vi "Test Case Description Reset on Test Start.vi"(8 "error in (no error)":errorcluster, 11 "Result Model Result Recording Test in":refnum<class "Result Model Result Recording Test.lvclass">) -> (0 "error out":errorcluster, 3 "Result Model Result Recording Test out":refnum<class "Result Model Result Recording Test.lvclass">)   [LabVIEW 2020, in "Result Model Result Recording Test.lvclass"]
uses:
  Result Model Result Recording Test.lvclass
  source/Core/Result/Type.ctl
  source/Core/Result/Result.lvlib
  source/Core/Result/Status.ctl
  source/Core/Result/Result.ctl
  ae2c71b8-32bb-49d1-8500-0119bfec74ff.vi
  source/User Interface/Result Model/Result Model.lvclass
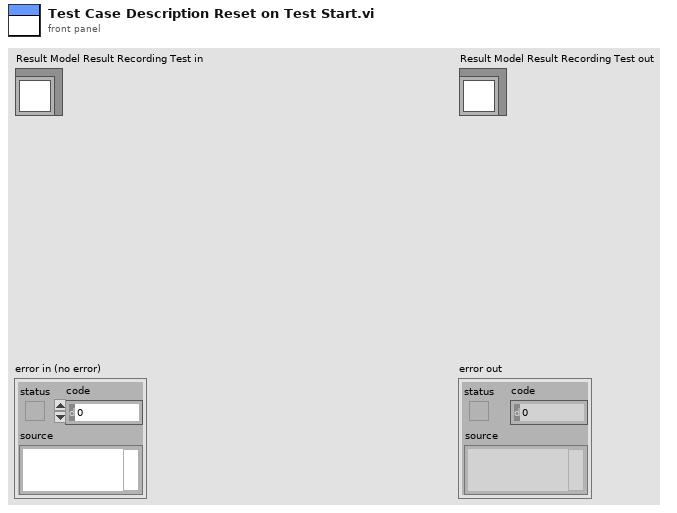
[diagram p1: front panel]
types:
  T1 = typedef "Result.lvlib/Result.ctl" = cluster{"Name":string, "Description":string, "Status":T2, "Result Type":T3, "Execution Time":dbl, "Data":cluster{"Expected":variant, "Actual":variant, "Delta":variant}}
  T2 = typedef "Result.lvlib/Status.ctl" = enum16{"", "Passed", "Failed", "Error", "Skipped", "Setup Error", "Broken", "Teardown Error"}
  T3 = typedef "Result.lvlib/Type.ctl" = enum16{"Test Case", "Test Suite", "Test Run", "Pass", "Fail", "Skip", "Pass if", "Fail if", "Pass if Error", "Fail if Error", "Pass if Equal", "Fail if Equal"}
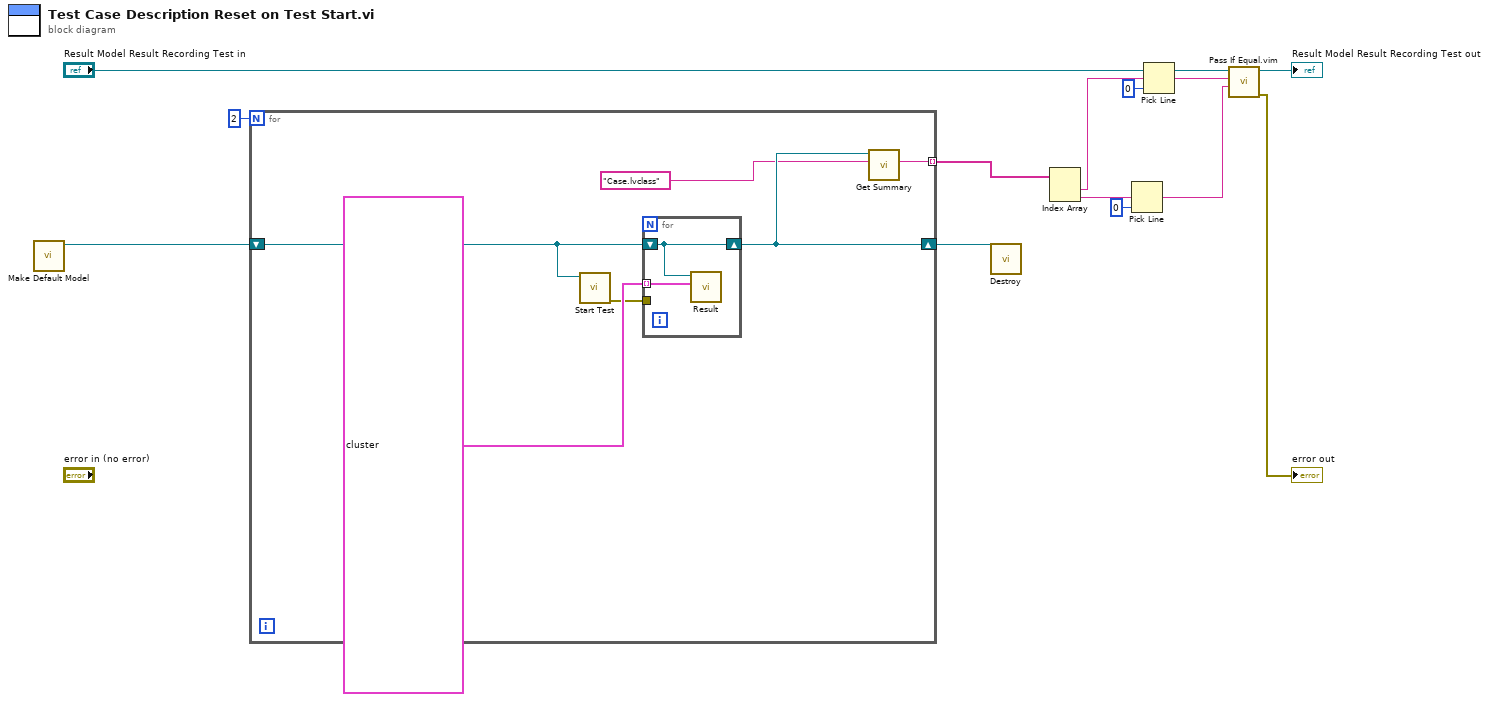
[diagram p0: block diagram]
diagram:
  n1 = call "Make Default Model.vi"() -> ("Result Model out"=w13:refnum<class "Result Model.lvclass">)  [unwired: 10 in, 1 out]
  n2 = for {
    N: 2 -> [_]
    shift-right: [w18] -> w8
    shift-left: w13 -> [w14]
    tunnel: [w17] -> w7 mode=indexing
    n3 = call "Start Test.vi"("Result Model by Reference In"=w14) -> ("error out"=w15:errorcluster)  [unwired: 10 in]
    n4 = for {
      tunnel: T1[] [{"Name"="Case.lvclass:Test Method.vi", "Description"="Failed:\nMessage", "Status"=enum."Failed", "Result Type"=enum."Pass", "Execution Time"=0.107, "Data"={"Expected"=variant, "Actual"=variant, "Delta"=variant}}, {"Name"="Case.lvclass:Test Method.vi", "Description"="", "Status"=enum."Passed", "Result Type"=enum."Test Case", "Execution Time"=0.0, "Data"={"Expected"=variant, "Actual"=variant, "Delta"=variant}}] ("Results") -> [w21] mode=indexing
      shift-right: [w20] -> w18
      shift-left: w14 -> [w20]
      tunnel: w15 -> [_]
      n5 = call-dynamic "Result.vi"("Results"=w21, "Result Model by Reference In"=w20) -> ()  [unwired: 9 in, 1 out]
    }
    n6 = call "Get Summary.vi"("Item"="Case.lvclass", "Result Model by Reference In"=w18) -> ("Summary"=w17:string)  [unwired: 8 in, 1 out]
  }
  n7 = call "Destroy.vi"("Result Model in"=w8) -> ()  [unwired: 10 in, 1 out]
  n8 = Index Array(array=w7) -> (element #1=w6:string, element #2=w5:string)  [unwired: 2 in]
  n9 = Pick Line(multi-line string=w5, line index=0) -> (output string=w3:string)  [unwired: 1 in]
  n10 = Pick Line(multi-line string=w6, line index=0) -> (output string=w4:string)  [unwired: 1 in]
  n11 = call "Pass If Equal.vim"("Actual"=w3, "Expected"=w4, "LUnit Test Case In"="Result Model Result Recording Test in") -> ("error out"=→"error out":errorcluster, "LUnit Test Case Out"=→"Result Model Result Recording Test out":refnum<class "Result Model Result Recording Test.lvclass">)  [unwired: 7 in]
